vi "get uart settings.vi"(8 "error in (no error)":errorcluster, 10 "uart_settings":cluster{"Speed":u32, "UARTSetupFlags":u32}, 11 "id":i32) -> (0 "error out":errorcluster, 2 "uart_settings out":cluster{"Speed":u32, "UARTSetupFlags":u32}, 3 "function return":i32)   [LabVIEW 2012, in "libximc.lvlib"]
doc: "result_t XIMC_API get_uart_settings (device_t id, uart_settings_t* uart_settings);"
uses:
  libximc.lvlib
  libximc.dll
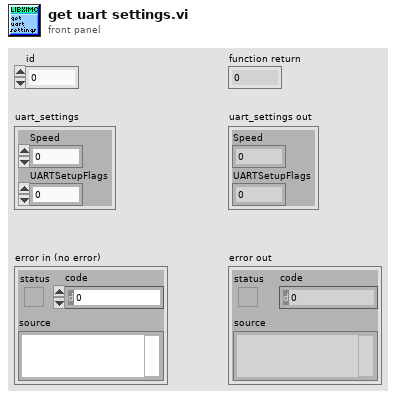
[diagram p1: front panel]
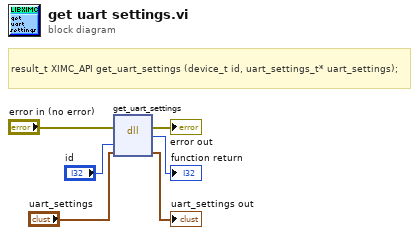
[diagram p0: block diagram]
diagram:
  # "result_t XIMC_API get_uart_settings (device_t id, uart_settings_t* uart_settings);"
  n1 = dll-call lib="E:/labview-2.12.1-Labview_12.0/ximcLVx32/libximc.*" fn="get_uart_settings"(error in="error in (no error)", "id"="id", "uart_settings"="uart_settings") -> (error out=→"error out":errorcluster, →"function return":i32, "uart_settings"=→"uart_settings out":cluster{"Speed":u32, "UARTSetupFlags":u32})  [unwired: 3 in, 1 out]
